vi "EnviraCom Decode Main.vi"(8 "error in (no error)":errorcluster) -> (0 "error out":errorcluster)   [LabVIEW 2023]
uses:
  <vilib>/Utility/file.llb/Read Delimited Spreadsheet (string).vi
panel:
  in  "Tab Control":enum32{"Page 1", "Page 2"}(tab)
  out "PV Data":string[][](array[string])
  out "HEX Only":string[](array[string])
  out "all rows":string[][](array[string])
  in  "file path (dialog if empty)":path
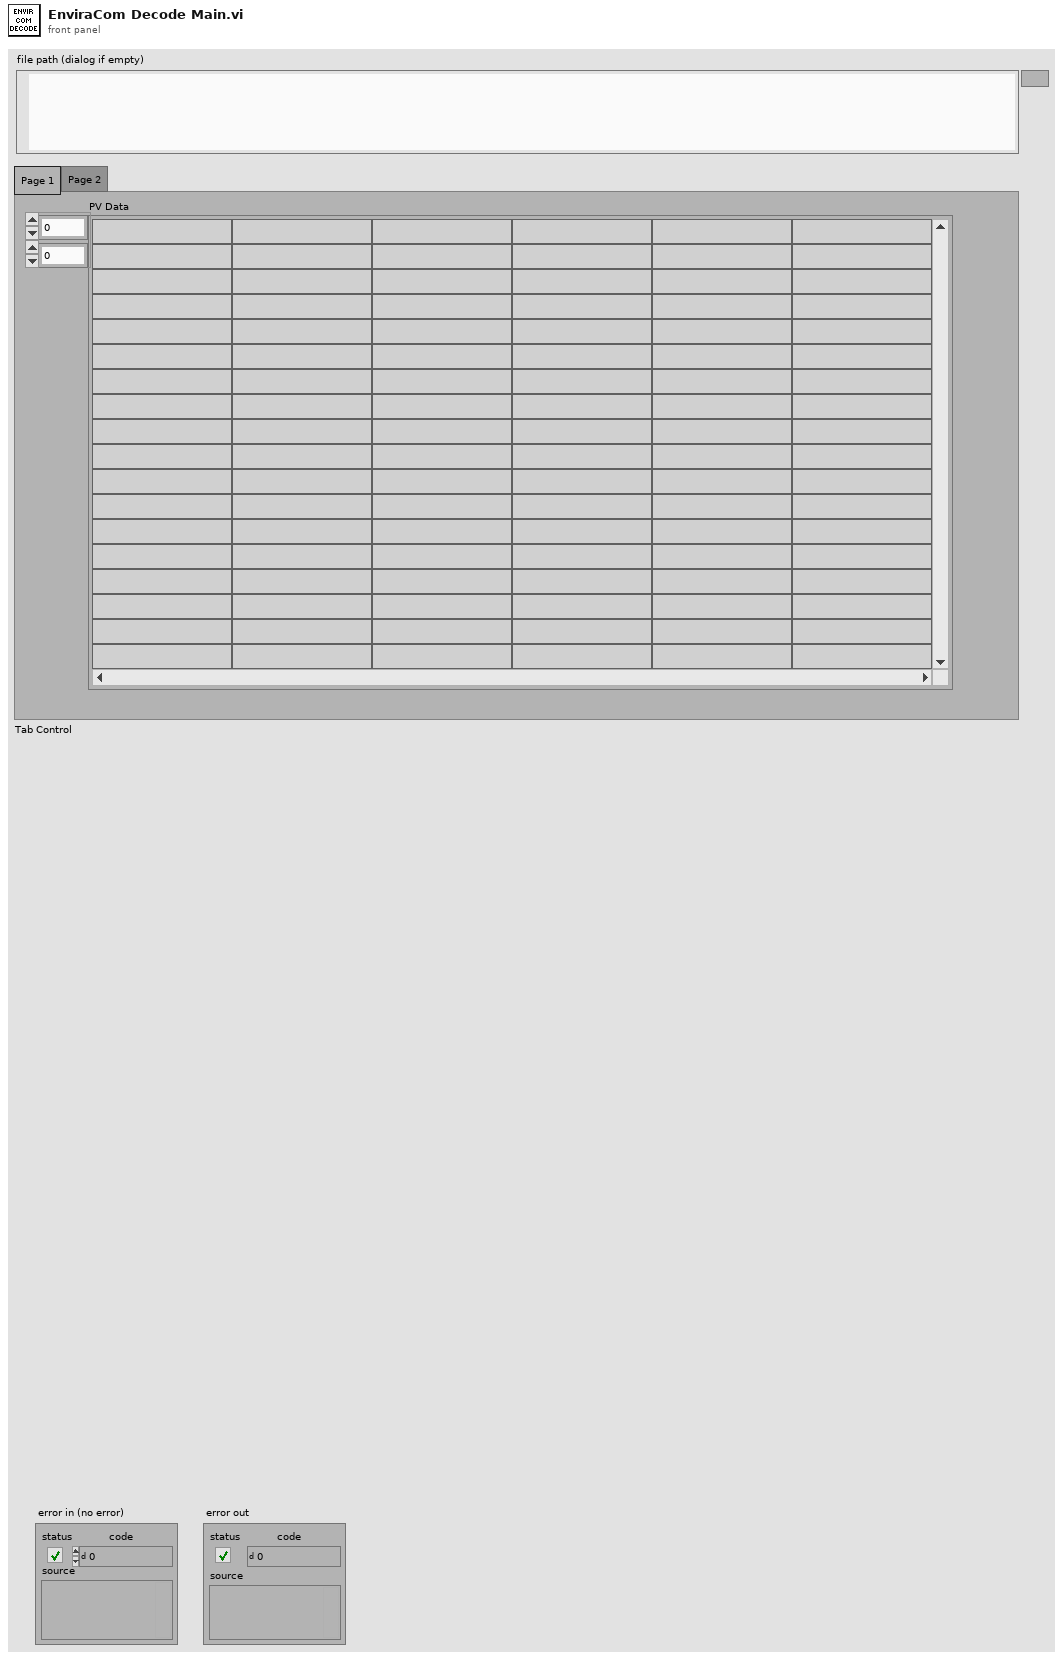
[diagram p1: front panel]
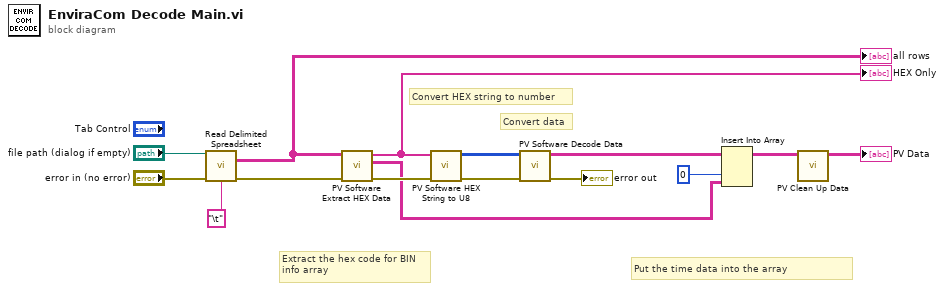
[diagram p0: block diagram]
diagram:
  # "Convert data"
  # "Convert HEX string to number"
  # "Extract the hex code for BIN\ninfo array"
  # "Put the time data into the array"
  n1 = call-poly <vilib>:"Read Delimited Spreadsheet.vi"("file path (dialog if empty)"="file path (dialog if empty)", "error in (no error)"="error in (no error)", "delimiter (\\t)"="\t" ("delimiter (\\t)")) -> ("all rows"=w13:string[][], "error out"=w8:errorcluster)  [unwired: 7 in, 4 out]
  "all rows" <- w13
  n2 = call "PV Software Extract HEX Data.vi"("error in (no error)"=w8, "All Data"=w13) -> ("error out"=w10:errorcluster, "Date and Time"=w4:string[][], "HEX Data (String)"=w11:string[])  [unwired: 7 in]
  "HEX Only" <- w11
  n3 = call "PV Software HEX String to U8.vi"("error in (no error)"=w10, "HEX Data (String)"=w11) -> ("error out"=w6:errorcluster, "HEX Data (U8)"=w12:u8[][])  [unwired: 8 in]
  n4 = call "PV Software Decode Data.vi"("error in (no error)"=w6, "HEX Data (U8)"=w12) -> ("error out"=→"error out":errorcluster, "PV Data"=w5:string[][])  [unwired: 8 in]
  n5 = Insert Into Array(array=w5, index (col)=0 ("disabled index (col)"), new element=w4) -> (w2:string[][])  [unwired: 1 in]
  n6 = call "PV Clean Up Data.vi"("PV Data in"=w2) -> ("PV Data out"=→"PV Data":string[][])  [unwired: 10 in]
